vi "jsonClose.vi"(8 "error in (no error)":errorcluster, 11 "d":i64) -> (0 "error out":errorcluster)   [LabVIEW 2015, in "rapidjson wrapper.lvlib"]
uses:
  rapidjson wrapper.lvlib
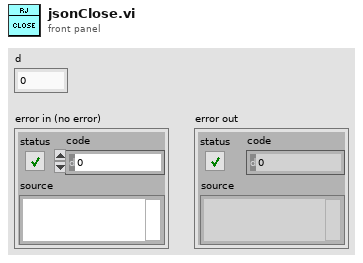
[diagram p1: front panel]
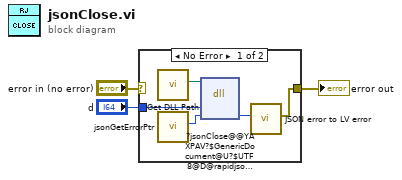
[diagram p0: block diagram]
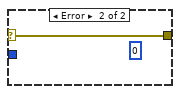
[diagram p2: hidden frame]
diagram:
  n1 = case shown="No Error" "error in (no error)" {
    selector: "error in (no error)" -> [_ w9]
    tunnel: [w5 w9] -> w3
    tunnel: "d" -> [w4 _]
    frame No Error {
      n2 = call "Get DLL Path.vi"() -> ("Path"=w8:path)  [unwired: 11 in]
      n3 = call "jsonGetErrorPtr.vi"() -> ("return type"=w7:i64)  [unwired: 10 in, 1 out]
      n4 = dll-call lib="C:/Users/tblair/Documents/Git Projects/LVrapidjson core/lvrjs/Debug/lvrjs.dll" fn="?jsonClose@@YAXPAV?$GenericDocument@U?$UTF8@D@rapidjson@@V?$MemoryPoolAllocator@VCrtAllocator@rapidjson@@@2@VCrtAllocator@2@@rapidjson@@0@Z"(path in=w8, "d"=w4, "jsonError"=w7) -> ("jsonError"=w6:i64)  [unwired: 4 in, 2 out]
      n5 = call "JSON error to LV error.vi"("jsonError"=w6) -> ("error out"=w5:errorcluster)  [unwired: 10 in]
    }
    frame Error {
      (unwired) i64 0 ("return type")
    }
  }
  "error out" <- w3
